vi "Default Open Flags for Download.vi"() -> (0 "open flags":T1)   [LabVIEW 2020, in "NI_SFTP.lvlib"]
uses:
  <vilib>/net/SFTP/NI_SFTP.lvlib
  <vilib>/net/SFTP/API/Support/Open Flags.ctl
  <vilib>/net/SFTP/API/Support/Command/SSH_FXP_OPEN/SSH_FXP_OPEN.lvclass
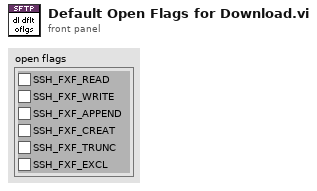
[diagram p1: front panel]
types:
  T1 = typedef "NI_SFTP.lvlib/SSH_FXP_OPEN.lvclass/Open Flags.ctl" = cluster{"SSH_FXF_READ":bool, "SSH_FXF_WRITE":bool, "SSH_FXF_APPEND":bool, "SSH_FXF_CREAT":bool, "SSH_FXF_TRUNC":bool, "SSH_FXF_EXCL":bool}
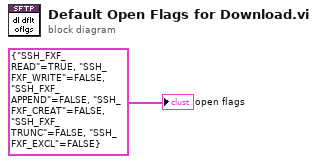
[diagram p0: block diagram]
diagram:
  "open flags" <- T1 {"SSH_FXF_READ"=TRUE, "SSH_FXF_WRITE"=FALSE, "SSH_FXF_APPEND"=FALSE, "SSH_FXF_CREAT"=FALSE, "SSH_FXF_TRUNC"=FALSE, "SSH_FXF_EXCL"=FALSE} ("open flags")
